vi "Test Module Broadcast Oscilloscope List.vi"(8 "error in (no error)":errorcluster, 11 "TestCase in":refnum<class "Test Module Init.lvclass">) -> (0 "error out":errorcluster, 3 "TestCase out":refnum<class "Test Module Init.lvclass">)   [LabVIEW 2020, in "Test Module Init.lvclass"]
uses:
  Test Module Init.lvclass
  <vilib>/addons/_JKI Toolkits/VI Tester/TestCase.llb/TestCase.lvclass
  Libraries/Osciloscope Tektronix/Osciloscope Tektronix.lvlib
  C:/Program Files (x86)/National Instruments/LabVIEW 2020/vi.lib/addons/_JKI Toolkits/VI Tester/TestCase.llb/TestCase.lvclass
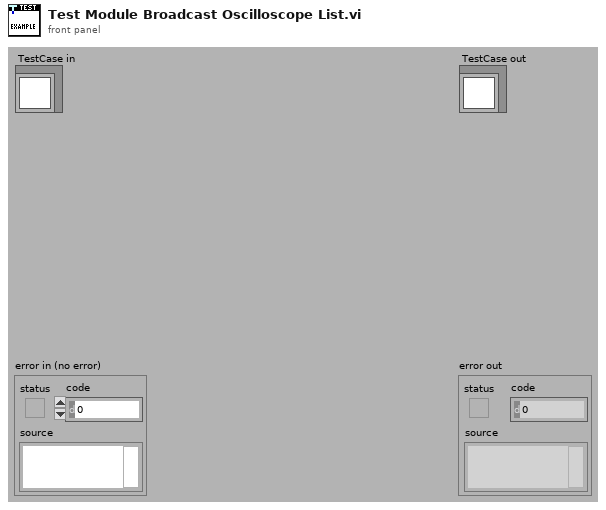
[diagram p1: front panel]
types:
  T1 = typedef "Osciloscope Tektronix.lvlib/Broadcast Events--cluster.ctl" = cluster{"Module Did Init":refnum<user-event>, "Status Updated":refnum<user-event>, "Error Reported":refnum<user-event>, "Module Did Stop":refnum<user-event>, "Update Module Execution Status":refnum<user-event>, "Oscilloscopes List":refnum<user-event>}
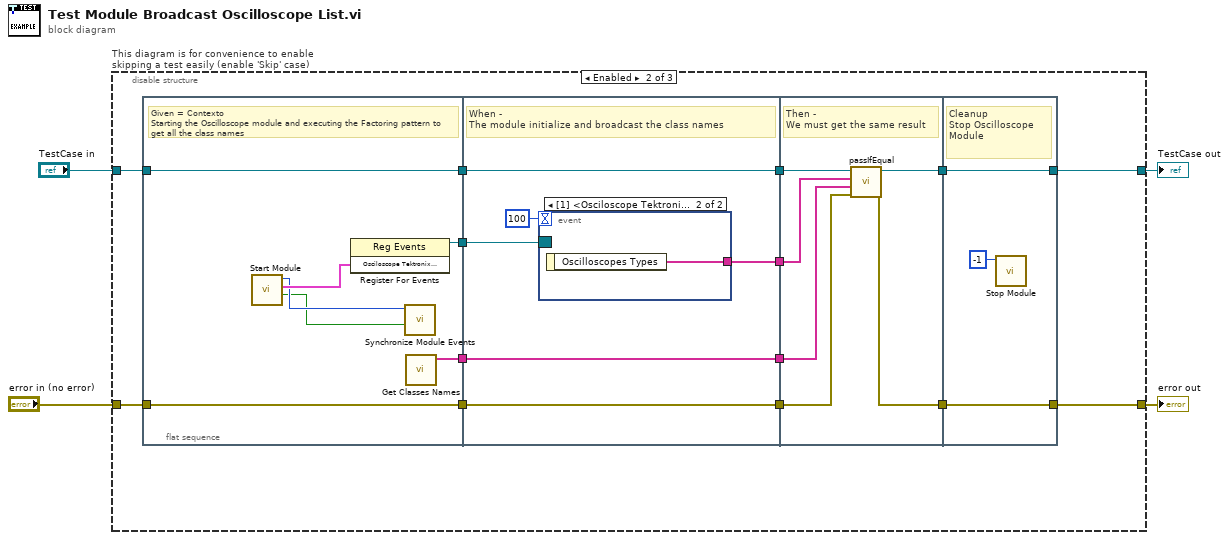
[diagram p0: block diagram]
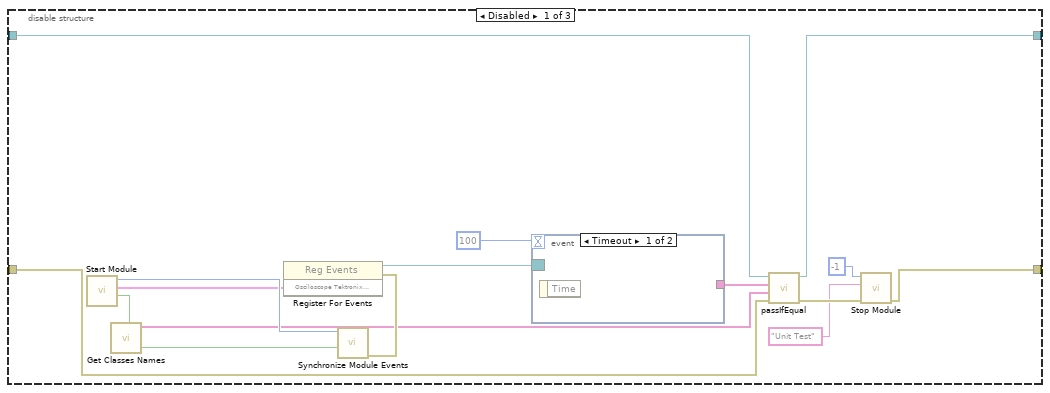
[diagram p2: hidden frame]
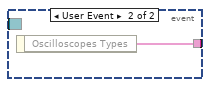
[diagram p3: hidden frame]
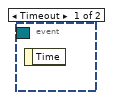
[diagram p4: hidden frame]
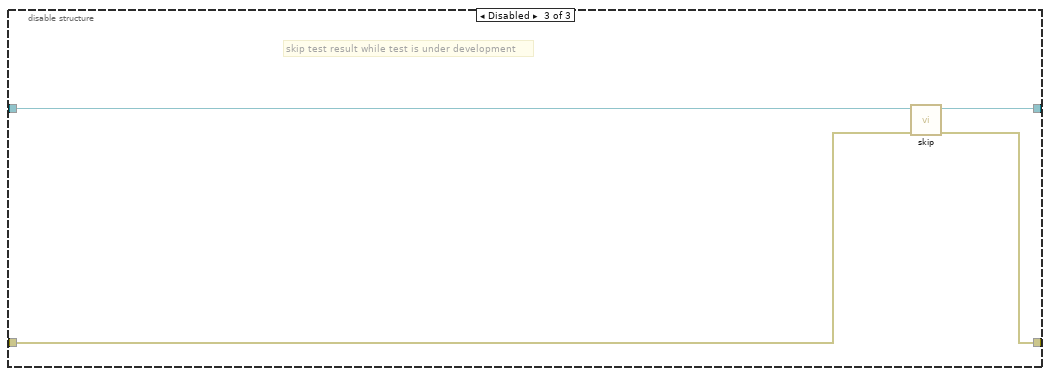
[diagram p5: hidden frame]
diagram:
  n1 = disable-structure "This diagram is for convenience to enable skipping a test easily (enable 'Skip' case)" shown="Enabled" {
    disable-tunnel: "TestCase in" -> [w19 w28 w61]
    disable-tunnel: [w18 w25 w59] -> w1
    disable-tunnel: [w8 w26 w60] -> w3
    disable-tunnel: "error in (no error)" -> [w17 w27 w58]
    frame Disabled {
      n2 = call "Start Module.vi"() -> ("Wait for Event Sync?"=w15:bool, "Osciloscope Tektronix Broadcast Events"=w14:T1, "Module ID"=w16:i32)  [unwired: 8 in, 1 out]
      n3 = call "Get Classes Names.vi"() -> ("Classes"=w11:string[])  [unwired: 11 in]
      n4 = register-events(w14) -> (reference out=w12:refnum<event-registration>, error out=w13:errorcluster)  [unwired: 2 in]
      n5 = call "Synchronize Module Events.vi"("error in"=w13, "Wait for Event Sync?"=w15, "Module ID in"=w16) -> ()  [unwired: 7 in, 2 out]
      n6 = event shown="[0] Timeout" {
        selector: w12 -> [_ _]
        dyn-events: _ -> [_ _]
        timeout: 100 -> [_ _]
        tunnel: [_ w20] -> w10
        event Timeout {
          n7 = event-data() -> ()  [unwired: 1 in, 1 out]
        }
        event User Event {
          n8 = event-data() -> ("Oscilloscopes Types"=w20:string[])  [unwired: 1 in]
        }
      }
      n9 = call-dynamic "passIfEqual.vi"("error in (no error)"=w17, "y"=w11, "x"=w10, "TestCase in"=w19) -> ("error out"=w7:errorcluster, "TestCase out"=w18:refnum<class "Test Module Init.lvclass">)  [unwired: 6 in]
      n10 = call "Stop Module.vi"("error in (no error)"=w7, "Origin"="Unit Test", "Module ID"=-1) -> ("error out"=w8:errorcluster)  [unwired: 8 in]
    }
    frame Enabled {
      n11 = flat-sequence {
        tunnel: w27 -> [w41]
        tunnel: [w40] -> w34
        tunnel: [w41] -> w33
        tunnel: w28 -> [w40]
        tunnel: [w36] -> w24
        tunnel: [w35] -> w23
        tunnel: [w47] -> w32
        tunnel: [w46] -> w31
        tunnel: w34 -> [w47]
        tunnel: w33 -> [w46]
        tunnel: w24 -> [w45]
        tunnel: w23 -> [w44]
        tunnel: [w44] -> w22
        tunnel: [w43] -> w21
        tunnel: [w53] -> w30
        tunnel: [w51] -> w29
        tunnel: w32 -> [w54]
        tunnel: w31 -> [w52]
        tunnel: w22 -> [w50]
        tunnel: w21 -> [w49]
        tunnel: [w57] -> w26
        tunnel: w30 -> [w56]
        tunnel: w29 -> [w57]
        tunnel: [w56] -> w25
        frame #0 {
          # "Given = Contexto\nStarting the Oscilloscope module and executing the Factoring pattern to get all the class names"
          n12 = call "Start Module.vi"() -> ("Wait for Event Sync?"=w37:bool, "Osciloscope Tektronix Broadcast Events"=w39:T1, "Module ID"=w38:i32)  [unwired: 8 in, 1 out]
          n13 = register-events(w39) -> (reference out=w36:refnum<event-registration>)  [unwired: 2 in, 1 out]
          n14 = call "Synchronize Module Events.vi"("Wait for Event Sync?"=w37, "Module ID in"=w38) -> ()  [unwired: 8 in, 2 out]
          n15 = call "Get Classes Names.vi"() -> ("Classes"=w35:string[])  [unwired: 11 in]
        }
        frame #1 {
          # "When -\nThe module initialize and broadcast the class names"
          n16 = event shown="[1] <Osciloscope Tektronix Broadcast Events.Oscilloscopes List>: User Event" {
            selector: w45 -> [_ _]
            dyn-events: _ -> [_ _]
            timeout: 100 -> [_ _]
            tunnel: [_ w48] -> w43
            event Timeout {
              n17 = event-data() -> ()  [unwired: 1 in, 1 out]
            }
            event User Event {
              n18 = event-data() -> ("Oscilloscopes Types"=w48:string[])  [unwired: 1 in]
            }
          }
        }
        frame #2 {
          # "Then -\nWe must get the same result"
          n19 = call-dynamic "passIfEqual.vi"("error in (no error)"=w52, "y"=w50, "x"=w49, "TestCase in"=w54) -> ("error out"=w51:errorcluster, "TestCase out"=w53:refnum<class "Test Module Init.lvclass">)  [unwired: 6 in]
        }
        frame #3 {
          # "Cleanup\nStop Oscilloscope Module"
          n20 = call "Stop Module.vi"("Module ID"=-1) -> ()  [unwired: 10 in, 1 out]
        }
      }
    }
    frame Disabled {
      # "skip test result while test is under development"
      n21 = call <vilib>:"skip.vi"("error in (no error)"=w58, "TestCase in"=w61) -> ("error out"=w60:errorcluster, "TestCase out"=w59:refnum<class "Test Module Init.lvclass">)  [unwired: 8 in]
    }
  }
  "error out" <- w3
  "TestCase out" <- w1
